vi "Lake Shore Cryotronics 340 Write Curve.vi"(3 "Array":dbl[](array[numeric])=[310.0, 61.21363], 4 "Write Curve\nHeader (F: Don't Write Header)":bool, 5 "index":dbl=91.0 format="%#_13g", 6 "error in (no error)":errorcluster, 7 "Curve (21)":dbl=21.0 min=21.0 max=60.0 step=1.0, 8 "String":string="ark 21 X86677 100 bbb 2\n0.25801\t4.45375E6\n0.27737\t2.62566E6\n0.29819\t1.60932E6\n0.32056\t1.02188E6\n0.34462\t670072.53973\n0.37048\t452436.26441\n0.39828\t313746.29687\n0.42817\t222930.45266\n0.4603\t161962.57325\n0.49484\t120085.41205\n0.53198\t90709.71558\n0.5719\t69700.59447\n0.61482\t54404.56821\n0.66096\t43083.06528\n0.71055\t34574.75489\n0.76388\t28089.82505\n0.8212\t23082.06075\n0.88283\t19167.7648\n0.94908\t16073.44039\n1.0203\t13601.46108\n1.09686\t11607.18615\n1.17917\t9983.47778\n1.26766\t8650.07908\n1.36279\t7546.23042\n1.46506\t6625.47288\n1.575\t5851.94795\n1.69319\t5197.73327\n1.82026\t4640.90424\n1.95685\t4164.10967\n2.1037\t3753.51517\n2.26157\t3398.01249\n2.43128\t3088.6226\n2.61373\t2818.04165\n2.80988\t2580.29273\n3.02074\t2370.45687\n3.24742\t2184.46393\n3.49112\t2018.92875\n3.7531\t1871.02208\n4.03474\t1738.36829\n4.33752\t1618.96369\n4.66302\t1511.11116\n5.01295\t1413.36735\n5.38913\t1324.49994\n5.79355\t1243.45283\n6.22831\t1169.31762\n6.6957\t1101.31025\n7.19817\t1038.75164\n7.73834\t981.0517\n8.31905\t927.69602\n8.94333\t878.23474\n9.61446\t832.27325\n10.33596\t789.46439\n11.1116\t749.50181\n11.94545\t712.1145\n12.84187\t677.06201\n13.80556\t644.13049\n14.84156\t613.12931\n15.95532\t583.88816\n17.15265\t556.25465\n18.43983\t530.09215\n19.82361\t505.27808\n21.31123\t481.70232\n22.91048\t459.26597\n24.62975\t437.8802\n26.47804\t417.46531\n28.46502\t397.94989\n30.60112\t379.27007\n32.89751\t361.36896\n35.36624\t344.19602\n38.02022\t327.70658\n40.87336\t311.86138\n43.94061\t296.62609\n47.23804\t281.97099\n50.78292\t267.87048\n54.59381\t254.3027\n58.69068\t241.2492\n63.095\t228.69448\n67.82982\t216.62562\n72.91996\t205.0319\n78.39208\t193.90438\n84.27485\t183.23555\n90.59907\t173.01889\n97.39788\t163.24857\n104.70689\t153.91906\n112.56439\t145.02481\n121.01154\t136.55996\n130.09259\t128.51808\n139.8551\t120.89196\n150.35022\t113.6734\n161.63293\t106.85306\n173.76232\t100.42039\n186.80193\t94.36354\n200.82007\t88.66931\n215.89018\t83.32316\n232.09118\t78.30923\n249.50796\t73.61033\n268.23174\t69.20805\n288.36061\t65.08274\n310\t61.21363\n", 9 "VISA resource name":refnum<visa-resource-name>="GPIB0::11::INSTR") -> (0 "error out":errorcluster)   [LabVIEW 2014]
doc: "This vi was designed to demonstrate typical usage of sub vi's containing the 340 curve functions.\n\nThis vi performs 3 curve functions, write curve header, write curve point, and save curve to flash. A typical way to use this vi would be to first write a curve header, then write multiple curve points until all points are written. Finally, run the vi selecting the save curve to flash function. Curves are not saved in memory until the save curve to flash function."
uses:
  LANL/Libraries/Instruments/Vendor Supplied/Lake Shore Cryotronics 340/Lake Shore Cryotronics 340.lvlib
panel:
  in  "format string":string="%s%s%s%f%s%d"
  in  "Write Curve\nPoint (F: Don't Write Point)":bool
  in  "Header":T1={"Curve Name (\"\")"="arkady", "Curve Data Format (0: mV/K)"=2, "Curve Serial Number (\"\")"="", "Limit Value (0.000)"=0.0, "Temp\nCoefficient (0: Negative)"=1} {"Temp\nCoefficient (0: Negative)" items=["Negative", "Positive"]; "Limit Value (0.000)" min=0.0 max=1500.0 step=0.001 format="%.3f"; "Curve Data Format (0: mV/K)" items=["mV/K", "V/K", "Ohms/K", "Log Ohms/K", "Log Ohms/Log K"]}
  in  "Save Curve\nto Flash (T: Save Curve)":bool=TRUE
  # "Copyright 2005. National Instruments Corporation"
  # "Write Header\nDon't Write Header"
  # "Write Point\nDon't Write Point"
  # "Save Curve\nDon't Save Curve"
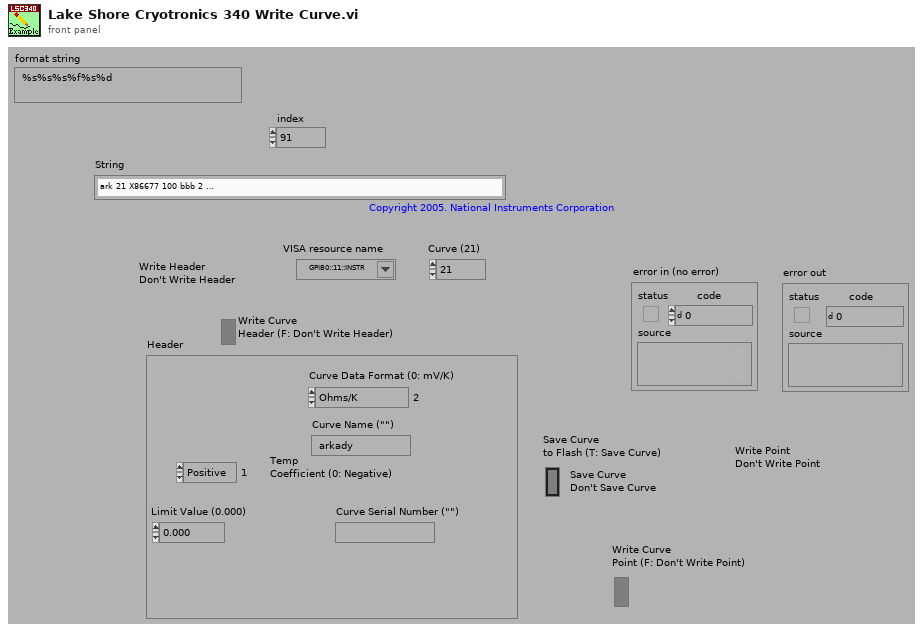
[diagram p1: front panel]
types:
  T1 = cluster{"Curve Name (\"\")":string, "Curve Data Format (0: mV/K)":u16, "Curve Serial Number (\"\")":string, "Limit Value (0.000)":dbl, "Temp\nCoefficient (0: Negative)":u16}
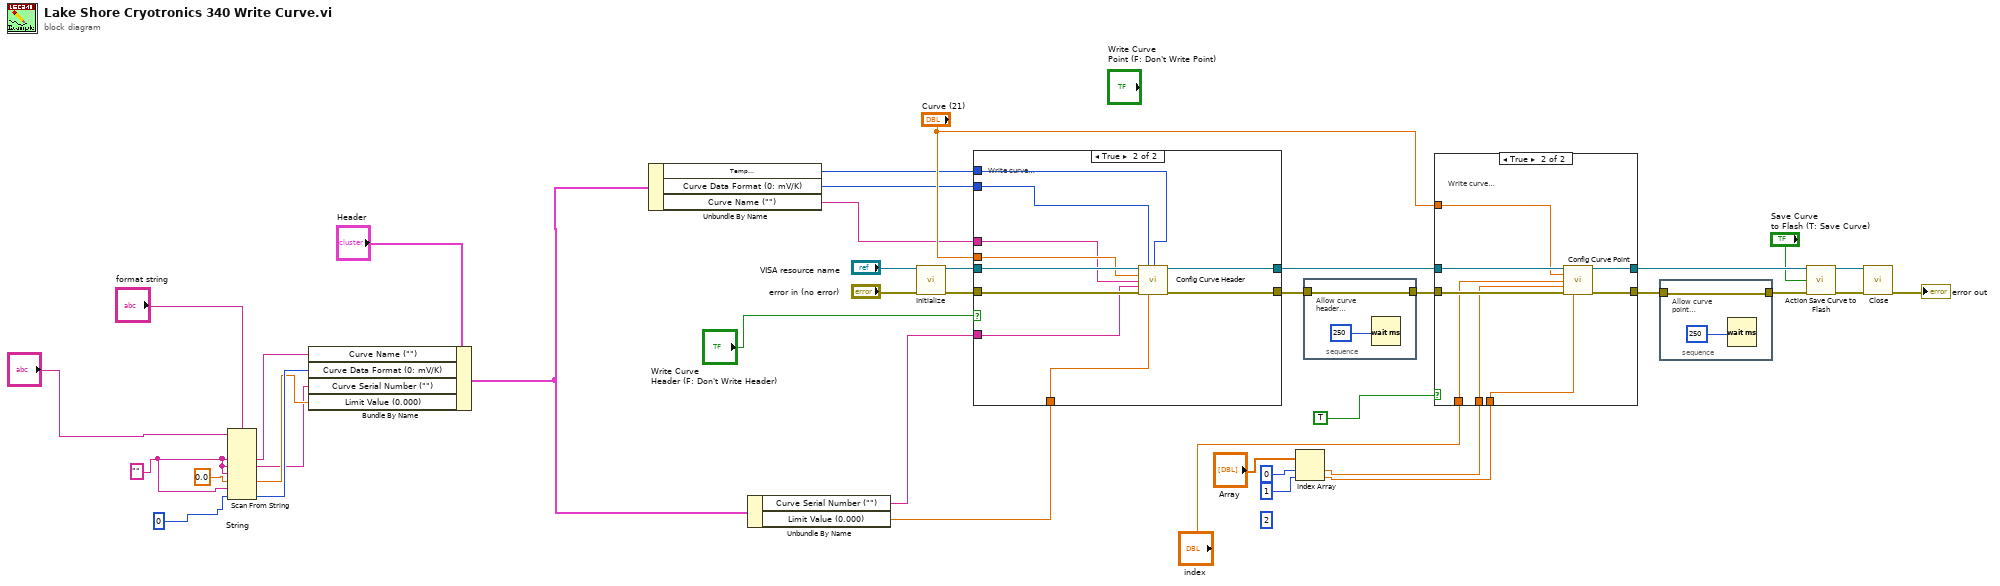
[diagram p0: block diagram]
diagram:
  w10 = "" ("String")
  (unwired) 2 ("index")
  n1 = Scan From String(format string="format string", input string="String", default 1=w10, default 2=w10, default 3=w10, default 4=0.0 ("default value 3"), default 5=w10, default 6=u16 0 ("Curve Data Format (0: mV/K)")) -> (output 1=w8:string, output 2=w5:string, output 4=w6:dbl, output 6=w7:u16)  [unwired: 4 in, 3 out]
  n2 = Bundle By Name(cluster="Header", "Curve Name (\"\")"=w8, "Curve Data Format (0: mV/K)"=w7, "Curve Serial Number (\"\")"=w5, "Limit Value (0.000)"=w6) -> (w14:T1)
  n3 = Unbundle By Name(w14) -> ("Temp\nCoefficient (0: Negative)"=w19:u16, "Curve Data Format (0: mV/K)"=w20:u16, "Curve Name (\"\")"=w23:string)
  n4 = Unbundle By Name(w14) -> ("Curve Serial Number (\"\")"=w22:string, "Limit Value (0.000)"=w21:dbl)
  n5 = call "Initialize.vi"("VISA resource name"="VISA resource name", "error in (no error)"="error in (no error)") -> ("VISA resource name out"=w28:refnum<visa-resource-name>, "error out"=w29:errorcluster)  [unwired: 3 in, 9 out]
  n6 = case shown="True" "Write Curve\nHeader (F: Don't Write Header)" {
    tunnel: w28 -> [w41 w51]
    tunnel: w29 -> [w40 w50]
    tunnel: [w41 w49] -> w39
    tunnel: [w40 w48] -> w35
    tunnel: "Curve (21)" -> [_ w47]
    tunnel: w23 -> [_ w46]
    tunnel: w22 -> [_ w45]
    tunnel: w21 -> [_ w44]
    tunnel: w20 -> [_ w43]
    tunnel: w19 -> [_ w42]
    frame False {
      # "Don't write curve header."
    }
    frame True {
      # "Write curve header."
      n7 = call "Config Curve Header.vi"("VISA resource name"=w51, "Curve Data Format (0: mV/K)"=w43, "Temp Coefficient (0: Negative)"=w42, "Curve (21)"=w47, "Curve Name (\"\")"=w46, "Curve Serial Number (\"\")"=w45, "error in (no error)"=w50, "Limit Value (0.000)"=w44) -> ("VISA resource name out"=w49:refnum<visa-resource-name>, "error out"=w48:errorcluster)  [unwired: 6 out]
    }
  }
  n8 = Index Array(array="Array", index #1=0 ("index"), index #2=1 ("index")) -> (element #1=w2:dbl, element #2=w1:dbl)
  n9 = stacked-sequence {
    tunnel: w35 -> [w52]
    tunnel: [w52] -> w34
    frame #0 {
      # "Allow curve header\nto process."
      n10 = Wait (ms)(milliseconds to wait=u32 250) -> ()  [unwired: 1 out]
    }
  }
  n11 = case shown="True" TRUE {
    tunnel: w39 -> [w55 w63]
    tunnel: w34 -> [w54 w62]
    tunnel: "Curve (21)" -> [_ w61]
    tunnel: [w55 w60] -> w37
    tunnel: [w54 w59] -> w33
    tunnel: w1 -> [_ w58]
    tunnel: w2 -> [_ w57]
    tunnel: "index" -> [_ w56]
    frame False {
      # "Don't Write curve point."
    }
    frame True {
      # "Write curve point."
      n12 = call "Config Curve Point.vi"("VISA resource name"=w63, "Curve (21)"=w61, "Index (1)"=w56, "Temperature \nValue (0.00000)"=w57, "error in (no error)"=w62, "Units Value (0.00000)"=w58) -> ("VISA resource name out"=w60:refnum<visa-resource-name>, "error out"=w59:errorcluster)  [unwired: 8 out]
    }
  }
  n13 = stacked-sequence {
    tunnel: w33 -> [w64]
    tunnel: [w64] -> w32
    frame #0 {
      # "Allow curve point\nto process."
      n14 = Wait (ms)(milliseconds to wait=u32 250) -> ()  [unwired: 1 out]
    }
  }
  n15 = call "Action Save Curve to Flash.vi"("VISA resource name"=w37, "Save Curve to Flash (T: Save)"="Save Curve\nto Flash (T: Save Curve)", "error in (no error)"=w32) -> ("VISA resource name out"=w27:refnum<visa-resource-name>, "error out"=w26:errorcluster)  [unwired: 11 out]
  n16 = call "Close.vi"("VISA resource name"=w27, "error in (no error)"=w26) -> ("error out"=→"error out":errorcluster)  [unwired: 13 out]
